vi "Do.vi"(8 "error in (no error)":errorcluster, 11 "Task Actor in":refnum<class "Task Actor.lvclass">) -> (0 "error out":errorcluster, 3 "Task Actor out":refnum<class "Task Actor.lvclass">)   [LabVIEW 2023, in "HAL GOOP4.lvlib" / "Task Actor.lvlib" / "Task Actor.lvclass"]
uses:
  Task Actor.lvclass
  <vilib>/ActorFramework/Actor/Actor.lvclass/Actor.ctl
  Task Actor.lvclass/Task Actor.ctl
  Task Base/Task Base.lvclass
  <vilib>/ActorFramework/Actor/Actor.lvclass
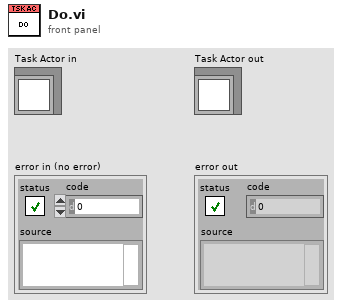
[diagram p1: front panel]
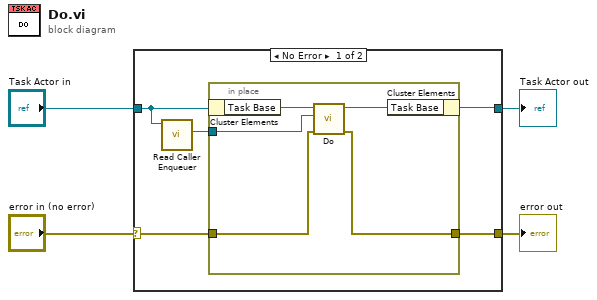
[diagram p0: block diagram]
diagram:
  n1 = case shown="No Error" "error in (no error)" {
    selector: "error in (no error)" -> [w9 w16]
    tunnel: [w8 w16] -> w3
    tunnel: [w7 w15] -> w1
    tunnel: "Task Actor in" -> [w6 w15]
    frame No Error {
      n2 = call <vilib>:"Read Caller Enqueuer.vi"("Actor"=w6) -> ("Caller Enqueuer"=w5:refnum<class "Message Enqueuer.lvclass">)  [unwired: 10 in]
      n3 = in-place {
        in-place-border: w9 -> [w13]
        in-place-border: [w12] -> w8
        in-place-border: w5 -> [w10]
        n4 = in-place-cluster #1(w6) -> ("Task Base"=w14:refnum<class "Task Base.lvclass">)
        n5 = call-dynamic "Do.vi"("error in"=w13, "Series Enqueuer"=w10, "Task Base in"=w14) -> ("error out"=w12:errorcluster, "Task Base out"=w11:refnum<class "Task Base.lvclass">)  [unwired: 7 in]
        n6 = in-place-cluster #1("Task Base"=w11) -> (w7:refnum<class "Task Actor.lvclass">)
      }
    }
    frame Error {
    }
  }
  "error out" <- w3
  "Task Actor out" <- w1
